vi "Unit Test - Backup Multiples of Size.vi"(8 "error in (no error)":errorcluster) -> (0 "error out":errorcluster)   [LabVIEW 2014]
uses:
  TableLogger_Actor/TableLoggerConfig.ctl
  TableLogger_Actor/TableLoggerTypes.ctl
  TableLogger_Actor/TableLoggerBackupConfig.ctl
  <vilib>/addons/_JKI Toolkits/Caraya/classes/Test/Test.lvclass
  TableLogger_Actor/TableLogger_Actor.lvlib
panel:
  # "Connector Pane"
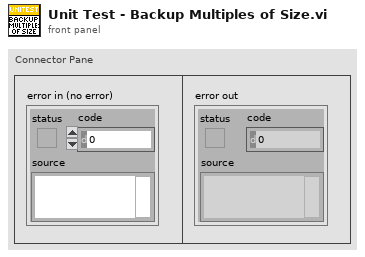
[diagram p1: front panel]
types:
  T1 = typedef "TableLogger_Actor.lvlib/TableLoggerConfig.ctl" = cluster{"TableLogger":T2, "DB File Path":path, "DB Backup Config":T3}
  T2 = typedef "TableLogger_Actor.lvlib/TableLoggerTypes.ctl" = enum16{"CSV Logger", "SQLite Logger"}
  T3 = typedef "TableLogger_Actor.lvlib/TableLoggerBackupConfig.ctl" = cluster{"Directory":path, "UTC Time Format":bool, "On Launch":bool, "Interval (Hours)":dbl, "Size Multiples (Bytes)":i32}
  T4 = typedef "TableLogger_Actor.lvlib/TableLoggerDataCluster.ctl" = cluster{"Numeric Data":i32, "Float Data":dbl, "String Data":string, "Enum Data":enum16{"Enum Item 1", "Enum Item 2"}, "Array Data":i32[]}
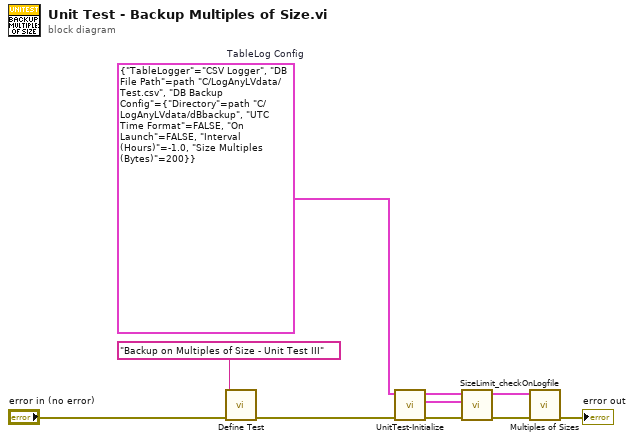
[diagram p0: block diagram]
diagram:
  w5 = T1 {"TableLogger"=enum."CSV Logger", "DB File Path"=path "C:/LogAnyLVdata/Test.csv", "DB Backup Config"={"Directory"=path "C:/LogAnyLVdata/dBbackup", "UTC Time Format"=FALSE, "On Launch"=FALSE, "Interval (Hours)"=-1.0, "Size Multiples (Bytes)"=200}}  # TableLog Config
  n1 = call <vilib>:"Define Test.vi"("error in (no error)"="error in (no error)", "Label (VI Title)"="Backup on Multiples of Size - Unit Test III") -> ("error out"=w6:errorcluster)  [unwired: 9 in]
  n2 = call "UnitTest-Initialize.vi"("error in"=w6, "Config IN"=w5) -> ("error out"=w4:errorcluster, "LV Data"=w1:T4, "Config OUT"=w2:T1)  [unwired: 7 in]
  n3 = call "SizeLimit_checkOnLogfile.vi"("error in"=w4, "LV Data"=w1, "Config IN"=w2) -> ("error out"=w3:errorcluster)  [unwired: 8 in]
  n4 = call "Multiples of Sizes.vi"("error in"=w3, "TableLogger Config"=w2) -> ("error out"=→"error out":errorcluster)  [unwired: 9 in]
